vi "Networking Enabled.vi"(11 "VolatusAPI in":refnum<class "VolatusAPI.lvclass">) -> (2 "Networking Enabled":bool, 3 "VolatusAPI out":refnum<class "VolatusAPI.lvclass">)   [LabVIEW 2020, in "Volatus.lvlib" / "VolatusAPI.lvclass"]
uses:
  VolatusAPI.lvclass
  VolatusAPI.lvclass/VolatusAPI.ctl
  lv-vecto/Vecto/Vecto/Vecto.lvclass
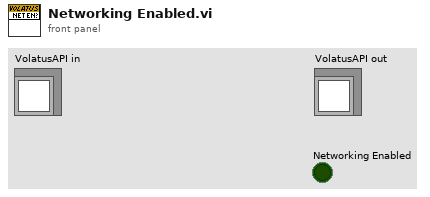
[diagram p1: front panel]
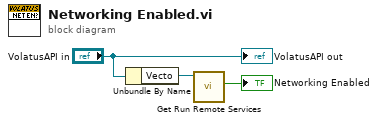
[diagram p0: block diagram]
diagram:
  n1 = Unbundle By Name("VolatusAPI in") -> ("Vecto"=w2:refnum<class "Vecto.lvclass">)
  n2 = call "Get Run Remote Services.vi"("Vecto in"=w2) -> ("Run Remote Services"=→"Networking Enabled":bool)  [unwired: 8 in, 2 out]
  "VolatusAPI out" <- "VolatusAPI in"
